vi "Radians to Degrees (Array EXT).vi"(3 "angles (rad)":ext[](array[numeric])) -> (1 "angles (deg)":ext[](array[numeric]))   [LabVIEW 2017, in "NI_AngleManipulation.lvlib"]
doc: "Converts a 1D array of angles from radians to degrees."
uses:
  <vilib>/Utility/AngleManip/NI_AngleManipulation.lvlib
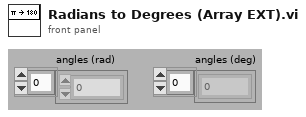
[diagram p1: front panel]
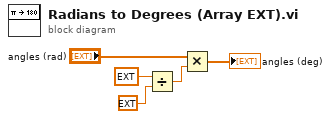
[diagram p0: block diagram]
diagram:
  n1 = Divide(x=ext 180.0 ("y"), y=ext 3.1415926535897932385) -> (x/y=w3:ext)
  n2 = Multiply(x="angles (rad)", y=w3) -> (x*y=→"angles (deg)":ext[])
